vi "Unpack control.vi"(8 "DRAM pack index init":T1, 9 "enable unpack":bool, 10 "input valid":bool, 11 "Data":T2) -> (0 "DRAM pack index out":T1, 1 "output valid?":bool, 3 "Unpacked data":u32)   [LabVIEW 2015]
uses:
  DRAM data index.ctl
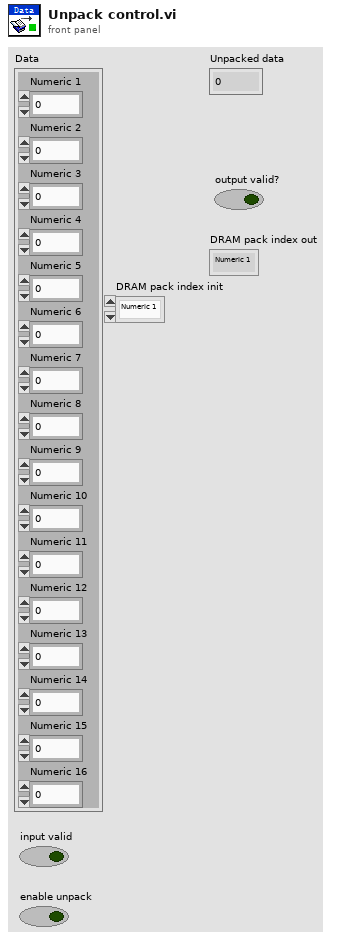
[diagram p1: front panel]
types:
  T1 = typedef "DRAM data index.ctl" = enum16{"Numeric 1", "Numeric 2", "Numeric 3", "Numeric 4", "Numeric 5", "Numeric 6", "Numeric 7", "Numeric 8", "Numeric 9", "Numeric 10", "Numeric 11", "Numeric 12", "Numeric 13", "Numeric 14", "Numeric 15", "Numeric 16"}
  T2 = cluster{"Numeric 1":u32, "Numeric 2":u32, "Numeric 3":u32, "Numeric 4":u32, "Numeric 5":u32, "Numeric 6":u32, "Numeric 7":u32, "Numeric 8":u32, "Numeric 9":u32, "Numeric 10":u32, "Numeric 11":u32, "Numeric 12":u32, "Numeric 13":u32, "Numeric 14":u32, "Numeric 15":u32, "Numeric 16":u32}
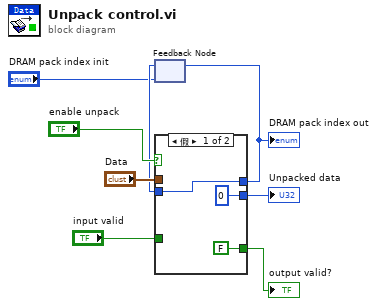
[diagram p0: block diagram]
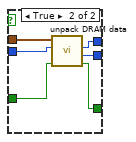
[diagram p2: hidden frame]
diagram:
  n1 = feedback #1("DRAM pack index init") -> (w2:T1)
  n2 = case shown="假" "enable unpack" {
    tunnel: "input valid" -> [_ w17]
    tunnel: "Data" -> [_ w16]
    tunnel: [u32 0 ("Galvo signal out") w15] -> w6
    tunnel: [w11 w13] -> w3
    tunnel: w2 -> [w11 w14]
    tunnel: [FALSE ("output valid?") w12] -> w8
    frame False {
    }
    frame True {
      n3 = call "unpack DRAM data.vi"("input valid?"=w17, "DRAM pack index in"=w14, "packer in"=w16) -> ("output valid?"=w12:bool, "Unpacked data"=w15:u32, "DRAM pack index out"=w13:T1)  [unwired: 5 in, 1 out]
    }
  }
  "DRAM pack index out" <- w3
  "output valid?" <- w8
  "Unpacked data" <- w6
  n4 = feedback-in #1(w3) -> ()
